vi "Reset Devices.vi"(0 "SLSC Local in":refnum<class "SLSC Local.lvclass">, 5 "devices":refnum<k21>="$DefaultDevices", 11 "error in (no error)":errorcluster) -> (4 "SLSC Local out":refnum<class "SLSC Local.lvclass">, 15 "error out":errorcluster)   [LabVIEW 2016, in "SLSC Interfaces.lvlib" / "SLSC Local.lvclass"]
uses:
  SLSC Local.lvclass
  <vilib>/SLSC/SLSC.lvlib
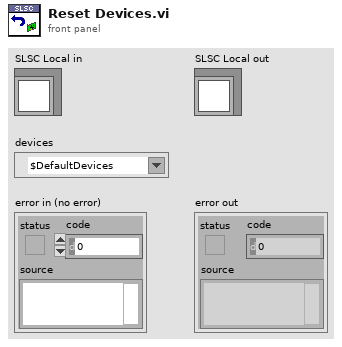
[diagram p1: front panel]
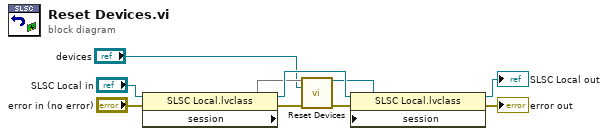
[diagram p0: block diagram]
diagram:
  n1 = property class="SLSC Local.lvclass"(reference="SLSC Local in", error in="error in (no error)") -> (reference out=w7:refnum<class "SLSC Local.lvclass">, error out=w9:errorcluster, "session"=w5)
  n2 = call <vilib>:"Reset Devices.vi"("session in"=w5, "devices"="devices", "error in (no error)"=w9) -> ("session out"=w4:refnum<k21>, "error out"=w8:errorcluster)  [unwired: 11 in]
  n3 = property class="SLSC Local.lvclass"(reference=w7, error in=w8, "session"=w4) -> (reference out=→"SLSC Local out":refnum<class "SLSC Local.lvclass">, error out=→"error out":errorcluster)
